vi "Request.vi"(8 "error in (no error)":errorcluster, 11 "Example Request in":refnum<k1>) -> (0 "error out":errorcluster)   [LabVIEW 2018]
uses:
  Example-Request.ctl
  Example-Reply.ctl
  Actor.lvclass
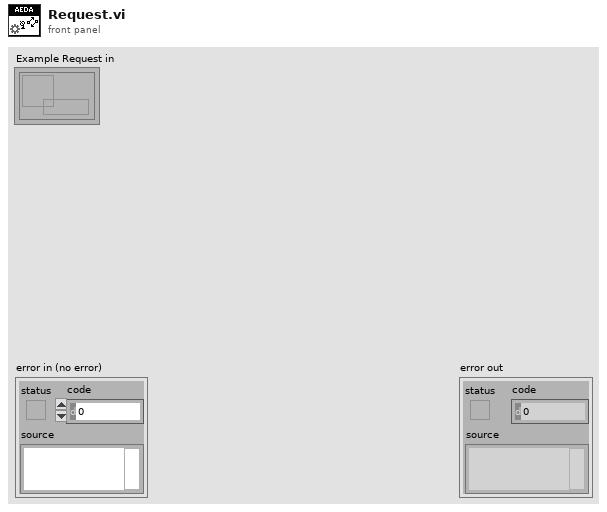
[diagram p1: front panel]
types:
  T1 = typedef "Actor.lvclass/Example-Request.ctl" = cluster{"Number":bool, "String":string}
  T2 = cluster{"Example-Request":refnum<user-event>, "event data":cluster{"Number":T1, "Reply":refnum<user-event>}}
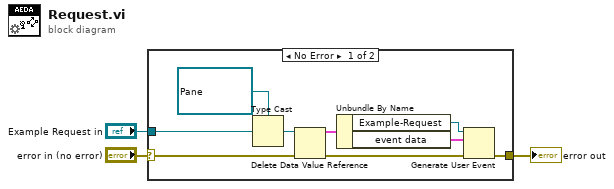
[diagram p0: block diagram]
diagram:
  n1 = case shown="No Error" "error in (no error)" {
    selector: "error in (no error)" -> [w9 w13]
    tunnel: [w4 w13] -> w2
    tunnel: "Example Request in" -> [w12 _]
    frame No Error {
      n2 = Type Cast(type=refnum<data-value> refnum ("data value reference"), x=w12) -> (*(type *) &x=w10:refnum<data-value>)
      n3 = Delete Data Value Reference(data value reference=w10, error in=w9) -> (data value=w8:T2, error out=w5:errorcluster)
      n4 = Unbundle By Name(w8) -> ("Example-Request"=w7:refnum<user-event>, "event data"=w6:cluster{"Number":T1, "Reply":refnum<user-event>})
      n5 = Generate User Event(user event=w7, event data cluster=w6, error in=w5) -> (error out=w4:errorcluster)  [unwired: 1 in, 1 out]
    }
    frame Error {
    }
  }
  "error out" <- w2
